vi "Set MB session in.vi"(10 "MB Serial Master:MB_Master":refnum<class "MB_Master.lvclass">, 11 "THM-V6数字型温湿度 in":refnum<class "THM-V6数字型温湿度.lvclass">) -> (3 "THM-V6数字型温湿度 out":refnum<class "THM-V6数字型温湿度.lvclass">)   [LabVIEW 2016, in "THM-V6数字型温湿度.lvlib" / "THM-V6数字型温湿度.lvclass"]
uses:
  <vilib>/Plasmionique/MB Master/MB_Master/MB_Master.lvclass
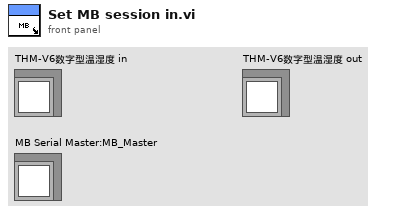
[diagram p1: front panel]
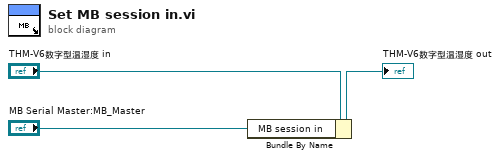
[diagram p0: block diagram]
diagram:
  n1 = Bundle By Name(cluster="THM-V6数字型温湿度 in", "MB session in"="MB Serial Master:MB_Master") -> (→"THM-V6数字型温湿度 out":refnum<class "THM-V6数字型温湿度.lvclass">)
